vi "Legendre Polynomial_Normalized (1D).vi"(8 "m":i32, 9 "n":i32, 11 "X":dbl[](array[numeric])) -> (3 "Nnm(X)":dbl[](array[numeric]))   [LabVIEW 2017, in "NI_AAL_Polynomial.lvlib"]
uses:
  <vilib>/Analysis/NI_AAL_Polynomial.lvlib
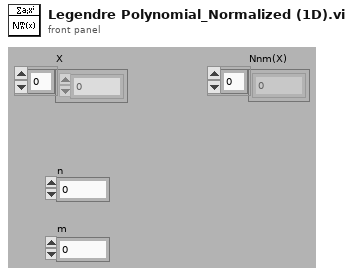
[diagram p1: front panel]
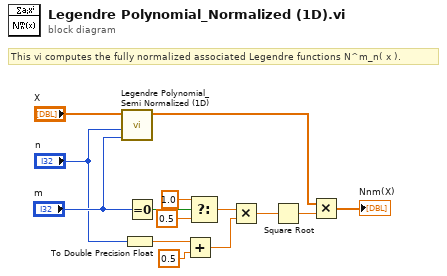
[diagram p0: block diagram]
diagram:
  # "This vi computes the fully normalized associated Legendre functions N^m_n( x )."
  n1 = call <vilib>:"Legendre Polynomial_Semi Normalized (1D).vi"("m"="m", "n"="n", "X"="X") -> ("Snm(X)"=w4:dbl[])  [unwired: 8 out]
  n2 = To Double Precision Float(number="n") -> (double precision float=w8:dbl)
  n3 = Equal To 0?(x="m") -> (x = 0?=w13:bool)
  n4 = Add(x=w8, y=0.5 ("x")) -> (x+y=w3:dbl)
  n5 = Select(t=1.0 ("f"), s=w13, f=0.5) -> (s? t:f=w12:dbl)
  n6 = Multiply(x=w12, y=w3) -> (x*y=w6:dbl)
  n7 = Square Root(x=w6) -> (sqrt(x)=w5:dbl)
  n8 = Multiply(x=w4, y=w5) -> (x*y=→"Nnm(X)":dbl[])
